vi "Monitor Acceleration.vi"(8 "error in (no error)":errorcluster, 9 "Y-Axis In":refnum<class "iMotion Controller.lvclass">, 10 "X-Axis In":refnum<class "iMotion Controller.lvclass">, 11 "Stage Data Class":refnum<data-value>) -> (0 "error out":errorcluster, 1 "Y-Axis Out":refnum<class "iMotion Controller.lvclass">, 2 "X-Axis Out":refnum<class "iMotion Controller.lvclass">, 3 "Stage Data Class":refnum<data-value>)   [LabVIEW 2022 SP3, in "XY Stage Process.lvlib" / "XY Stage Process.lvclass"]
uses:
  XY Stage Process.lvclass
  6046c730-44da-4461-abcf-74f1f8a9aa6a.vi
  XY Stage Data Class/Acceleration.ctl
  XY Stage Data Class/XY Stage Data Class.lvclass
  Axis Objects/iMotion Controller/iMotion Controller.lvclass
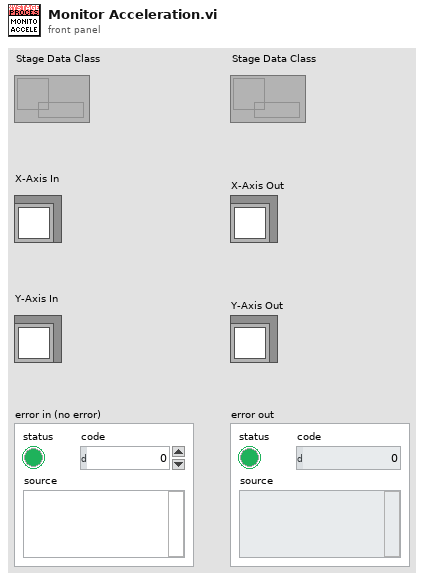
[diagram p1: front panel]
types:
  T1 = typedef "XY Stage Data Class.lvclass/Acceleration.ctl" = cluster{"X Acceleration":dbl, "Y Acceleration":dbl}
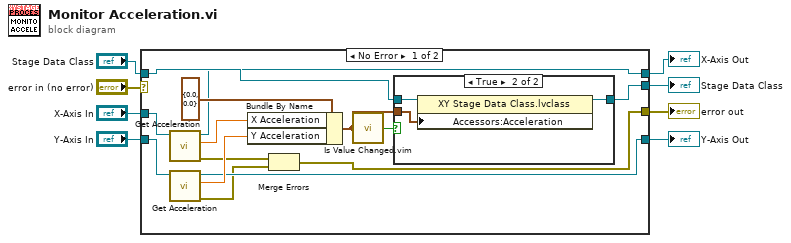
[diagram p0: block diagram]
diagram:
  n1 = case shown="No Error" "error in (no error)" {
    selector: "error in (no error)" -> [_ w27]
    tunnel: "Y-Axis In" -> [w15 w28]
    tunnel: "X-Axis In" -> [w16 w29]
    tunnel: "Stage Data Class" -> [w21 w30]
    tunnel: [w20 w30] -> w4
    tunnel: [w14 w29] -> w3
    tunnel: [w11 w28] -> w2
    tunnel: [w19 w27] -> w1
    frame No Error {
      n2 = call-dynamic "Get Acceleration.vi"("iMotion Controller in"=w16) -> ("error out"=w10:errorcluster, "Acceleration"=w13:dbl, "iMotion Controller out"=w14:refnum<class "iMotion Controller.lvclass">)  [unwired: 8 in]
      n3 = call-dynamic "Get Acceleration.vi"("iMotion Controller in"=w15) -> ("error out"=w9:errorcluster, "Acceleration"=w12:dbl, "iMotion Controller out"=w11:refnum<class "iMotion Controller.lvclass">)  [unwired: 8 in]
      n4 = Bundle By Name(cluster=T1 {"X Acceleration"=0.0, "Y Acceleration"=0.0} ("Acceleration"), "X Acceleration"=w13, "Y Acceleration"=w12) -> (w18:T1)
      n5 = Merge Errors(w10, w9) -> (w19:errorcluster)
      n6 = call "Is Value Changed.vim"("value"=w18) -> ("changed or first call?"=w22:bool)
      n7 = case shown="True" w22 {
        tunnel: [w23 w26] -> w20
        tunnel: w21 -> [w23 w25]
        tunnel: w18 -> [_ w24]
        frame False {
        }
        frame True {
          n8 = property class="XY Stage Data Class.lvclass"(reference=w25, "Accessors:Acceleration"=w24) -> (reference out=w26:refnum<data-value>)  [unwired: 1 in, 1 out]
        }
      }
    }
    frame Error {
    }
  }
  "Stage Data Class" <- w4
  "X-Axis Out" <- w3
  "Y-Axis Out" <- w2
  "error out" <- w1
